vi "Auto_Routine_RightTwoPieceThen2CenterTRAJ.vi"   [LabVIEW 2023]
uses:
  Shoulder/ShoulderGetSetpointEnum.ctl
  Trajectory/TrajectoryGlobals.vi
  <vilib>/Rock Robotics/WPI/ThirdParty/JAS_Junk/TrajLib/Trajectory_Library.lvlib
types:
  T1 = typedef "ShoulderGetSetpointEnum.ctl" = enum16{"ShoulderRest", "ShoulderSpeaker", "ShoulderAmp"}
  T2 = typedef "ShoulderGetSetpointEnum.ctl" = enum16{"ShoulderRest", "ShoulderShoot", "ShoulderAmp", "ArmFloorPickup", "ArmAmpDeposit", "ArmSpeakerShoot", "ArmStartPosition", "ArmRestPosition", "ArmSourceIntake", "ArmAwayShoot"}
  T3 = typedef "Trajectory_Library.lvlib/TRAJECTORY.ctl" = cluster{"TotalTImeSecs":dbl, "States":T4[]}
  T4 = typedef "Trajectory_Library.lvlib/TRAJ_STATE.ctl" = cluster{"TimeSeconds":dbl, "Velocity":dbl, "Acceleration":dbl, "POSE":T5, "Curvature":dbl}
  T5 = typedef "Trajectory_Library.lvlib/POSE2D.ctl" = cluster{"TRANSLATION":T6, "ROTATION":T7}
  T6 = typedef "Trajectory_Library.lvlib/TRANSLATION2D.ctl" = cluster{"X":dbl, "Y":dbl}
  T7 = typedef "Trajectory_Library.lvlib/ROTATION2D.ctl" = cluster{"VALUE":dbl, "COS":dbl, "SIN":dbl}
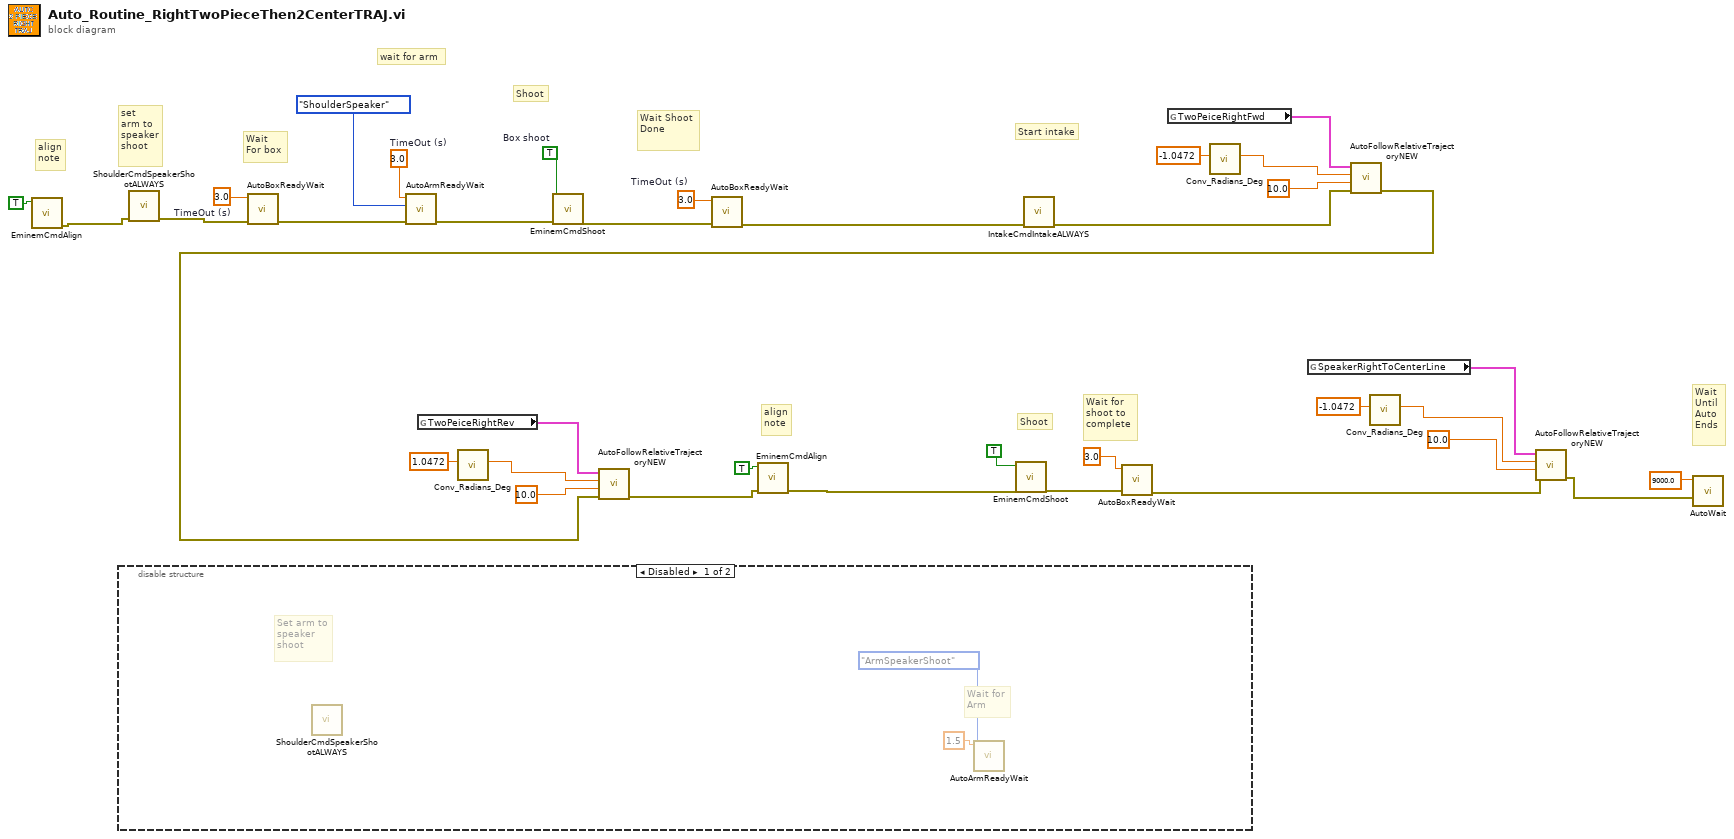
[diagram p0: block diagram]
diagram:
  w28 = 3.0  # TimeOut (s)
  w35 = TRUE  # Box shoot
  w34 = 3.0  # TimeOut (s)
  w31 = 3.0  # TimeOut (s)
  # "align\nnote"
  # "Wait\nUntil\nAuto \nEnds"
  # "Wait for\nshoot to\ncomplete"
  # "Shoot"
  # "Start intake"
  # "Wait Shoot\nDone"
  # "Shoot"
  # "Wait\nFor box"
  # "set \narm to\nspeaker\nshoot"
  # "align\nnote"
  # "wait for arm"
  n1 = call "EminemCmdAlign.vi"("box align"=TRUE) -> ("error out"=w29:errorcluster)  [unwired: 10 in]
  n2 = disable-structure shown="Disabled" {
    frame Disabled {
      # "Wait for\nArm"
      # "Set arm to\nspeaker \nshoot"
      n3 = call "ShoulderCmdSpeakerShootALWAYS.vi"() -> ()  [unwired: 11 in, 1 out]
      n4 = call "AutoArmReadyWait.vi"("ArmSetpoints"=ShoulderGetSetpointEnum."ArmSpeakerShoot", "TimeOut (s)"=1.5) -> ("error in (no error)"=w36:errorcluster)  [unwired: 8 in, 1 out]
    }
    frame Enabled {
    }
  }
  n5 = call "ShoulderCmdSpeakerShootALWAYS.vi"("error in (no error)"=w29) -> ("error out"=w27:errorcluster)  [unwired: 10 in]
  n6 = call "AutoBoxReadyWait.vi"("error in (no error)"=w27, "TimeOut (s)"=w28) -> ("error out"=w26:errorcluster)  [unwired: 9 in]
  n7 = call "AutoArmReadyWait.vi"("error in (no error)"=w26, "ArmSetpoints"=ShoulderGetSetpointEnum."ShoulderSpeaker", "TimeOut (s)"=w34) -> ("error out"=w32:errorcluster)  [unwired: 8 in]
  n8 = global read "TrajectoryGlobals.vi" "TwoPeiceRightRev"() -> (w17:T3)
  n9 = call <vilib>:"Conv_Radians_Deg.vi"("Radians"=1.0472) -> ("Degrees"=w15:dbl)  [unwired: 10 in]
  n10 = call "EminemCmdShoot.vi"("error in (no error)"=w32, "Box shoot"=w35) -> ("error out"=w33:errorcluster)  [unwired: 9 in]
  n11 = call "AutoBoxReadyWait.vi"("error in (no error)"=w33, "TimeOut (s)"=w31) -> ("error out"=w2:errorcluster)  [unwired: 9 in]
  n12 = call "IntakeCmdIntakeALWAYS.vi"("error in (no error)"=w2) -> ("error out"=w1:errorcluster)  [unwired: 10 in]
  n13 = global read "TrajectoryGlobals.vi" "TwoPeiceRightFwd"() -> (w25:T3)
  n14 = call <vilib>:"Conv_Radians_Deg.vi"("Radians"=-1.0472) -> ("Degrees"=w23:dbl)  [unwired: 10 in]
  n15 = global read "TrajectoryGlobals.vi" "SpeakerRightToCenterLine"() -> (w11:T3)
  n16 = call "AutoFollowRelativeTrajectoryNEW.vi"("error in (no error)"=w1, "TimeOut (s)"=10.0, "End Orientation"=w23, "Trajectory"=w25) -> ("error out"=w5:errorcluster)  [unwired: 7 in]
  n17 = call "AutoFollowRelativeTrajectoryNEW.vi"("error in (no error)"=w5, "TimeOut (s)"=10.0, "End Orientation"=w15, "Trajectory"=w17) -> ("error out"=w12:errorcluster)  [unwired: 7 in]
  n18 = call "EminemCmdAlign.vi"("error in (no error)"=w12, "box align"=TRUE) -> ("error out"=w4:errorcluster)  [unwired: 9 in]
  n19 = call "EminemCmdShoot.vi"("error in (no error)"=w4, "Box shoot"=TRUE) -> ("error out"=w20:errorcluster)  [unwired: 9 in]
  n20 = call "AutoBoxReadyWait.vi"("error in (no error)"=w20, "TimeOut (s)"=3.0) -> ("error out"=w7:errorcluster)  [unwired: 9 in]
  n21 = call <vilib>:"Conv_Radians_Deg.vi"("Radians"=-1.0472) -> ("Degrees"=w9:dbl)  [unwired: 10 in]
  n22 = call "AutoFollowRelativeTrajectoryNEW.vi"("error in (no error)"=w7, "TimeOut (s)"=10.0, "End Orientation"=w9, "Trajectory"=w11) -> ("error out"=w6:errorcluster)  [unwired: 7 in]
  n23 = call "AutoWait.vi"("error in (no error)"=w6, "TimeOut (s)"=9000.0) -> ()  [unwired: 9 in, 1 out]
